vi "Restarts by Flow Sandbox Original (FPGA).vi"() -> ()   [LabVIEW 2019]
uses:
  <vilib>/eio/EIONode/EIONode.xnode
  <vilib>/rvi/eio/common/nirviEmuTemplateMethod_errors.vi
  <vilib>/rvi/FXPMathLib/FxpMul/XNode/nifxpmath_Multiplier.xnode
  <vilib>/rvi/FXPMathLib/sim/FxpSim.dll
  <vilib>/Platform/TimedLoop/XDataNode/wakeup.ctl
  <vilib>/Platform/TimedLoop/XDataNode/XDNodeRunTimeDep.lvlib
  <vilib>/Platform/TimedLoop/XDataNode/nitl_modes.ctl
  <vilib>/Platform/TimedLoop/XDataNode/timing_clust.ctl
  <vilib>/Platform/TimedLoop/XDataNode/XDataNode.xnode
  <vilib>/rvi/Analysis/measure/dc-rms/XNode/niFpgaDC-RMS.xnode
  <vilib>/rvi/DataTransferAndStorage/Container/XNode/niFpgaContainer.xnode
  <vilib>/rvi/FXPMathLib/FxpAdd/XNode/nifxpmath_Add.xnode
  <userlib>/_NI SPI IP/FPGA/Controllers/Public/Spi Master Inputs.ctl
  <vilib>/eio/EIOMethodNode/EIOMethodNode.xnode
  Controls/SPI Channels.ctl
  <vilib>/rvi/FIFO/Fifo_Resource/niFpgaFifoEmulationRefIn.vi
  <vilib>/rvi/interface/RandomDataEmulation/nirviRandomDataFpgaReadWriteTemplate.vi
  <vilib>/rvi/FXPMathLib/basic elements/FxpIntAccumulator/simVIs/DllFxpIntAccumulator_sub.vi
  <vilib>/rvi/FXPMathLib/basic elements/FxpIntAccumulator/XNode/nifxpmath_IntAccumulator.xnode
  <vilib>/rvi/FXPMathLib/FxpSqrt/XNode/nifxpmath_Sqrt.xnode
  <vilib>/rvi/Analysis/common/codeGenErrors/XNode/niFpgaXNodeCodeGenErrorHandle.vi
  <vilib>/rvi/FXPMathLib/FxpSqrt/simVIs/DllSqrtTemp_sub.vi
  <vilib>/fxp/LVFixedPointOverflowPolicyTypeDef.ctl
  <vilib>/rvi/FXPMathLib/FxpSqrt/subVIs/nifxpmath_Sqrt_SimConfig.ctl
  <vilib>/rvi/FXPMathLib/basic elements/FxpIntAccumulator/subVIs/nifxpmath_IntAccumulator_SimConfig.ctl
  <vilib>/rvi/FXPMathLib/FxpSub/XNode/nifxpmath_Sub.xnode
  <vilib>/rvi/Memory/Memory_Emulation/nirvimemoryFastEmulation.vi
  <vilib>/rvi/Memory/Memory_Emulation/nirvimemoryEmulation.vi
  <userlib>/_NI SPI IP/FPGA/Controllers/Public/Transfer Settings.ctl
panel:
  in  "Pres/Flow":bool
  out "DetPres Starts":u32
  out "Pressure":fxp<+/-,28,17>
  out "Flow":fxp<+/-,28,17>
  out "Current":fxp<+/-,28,17>
  out "DetFlow Starts":u32
  in  "Position":i32
  in  "PreDataPts":i32=2000
  in  "Reset Restarts":bool
  in  "AI24-31 Data to Write":u64 format="%.0x"
  out "AI24-31":fxp<+/-,28,17>[](array[numeric])
  out "Read Data 2":u64 format="%.0x"
  in  "AI24-31 Settings":T1 {"Direction Change Bit" max=64 step=1; "Transfer Length (bits)" min=1 max=64 step=1}
  out "AI16-23":fxp<+/-,28,17>[](array[numeric])
  in  "AI16-23 Data to Write":u64 format="%.0x"
  out "Read Data":u64 format="%.0x"
  in  "AI16-23 Settings":T1 {"Direction Change Bit" max=64 step=1; "Transfer Length (bits)" min=1 max=64 step=1}
  in  "AO0":fxp<+/-,20,5>
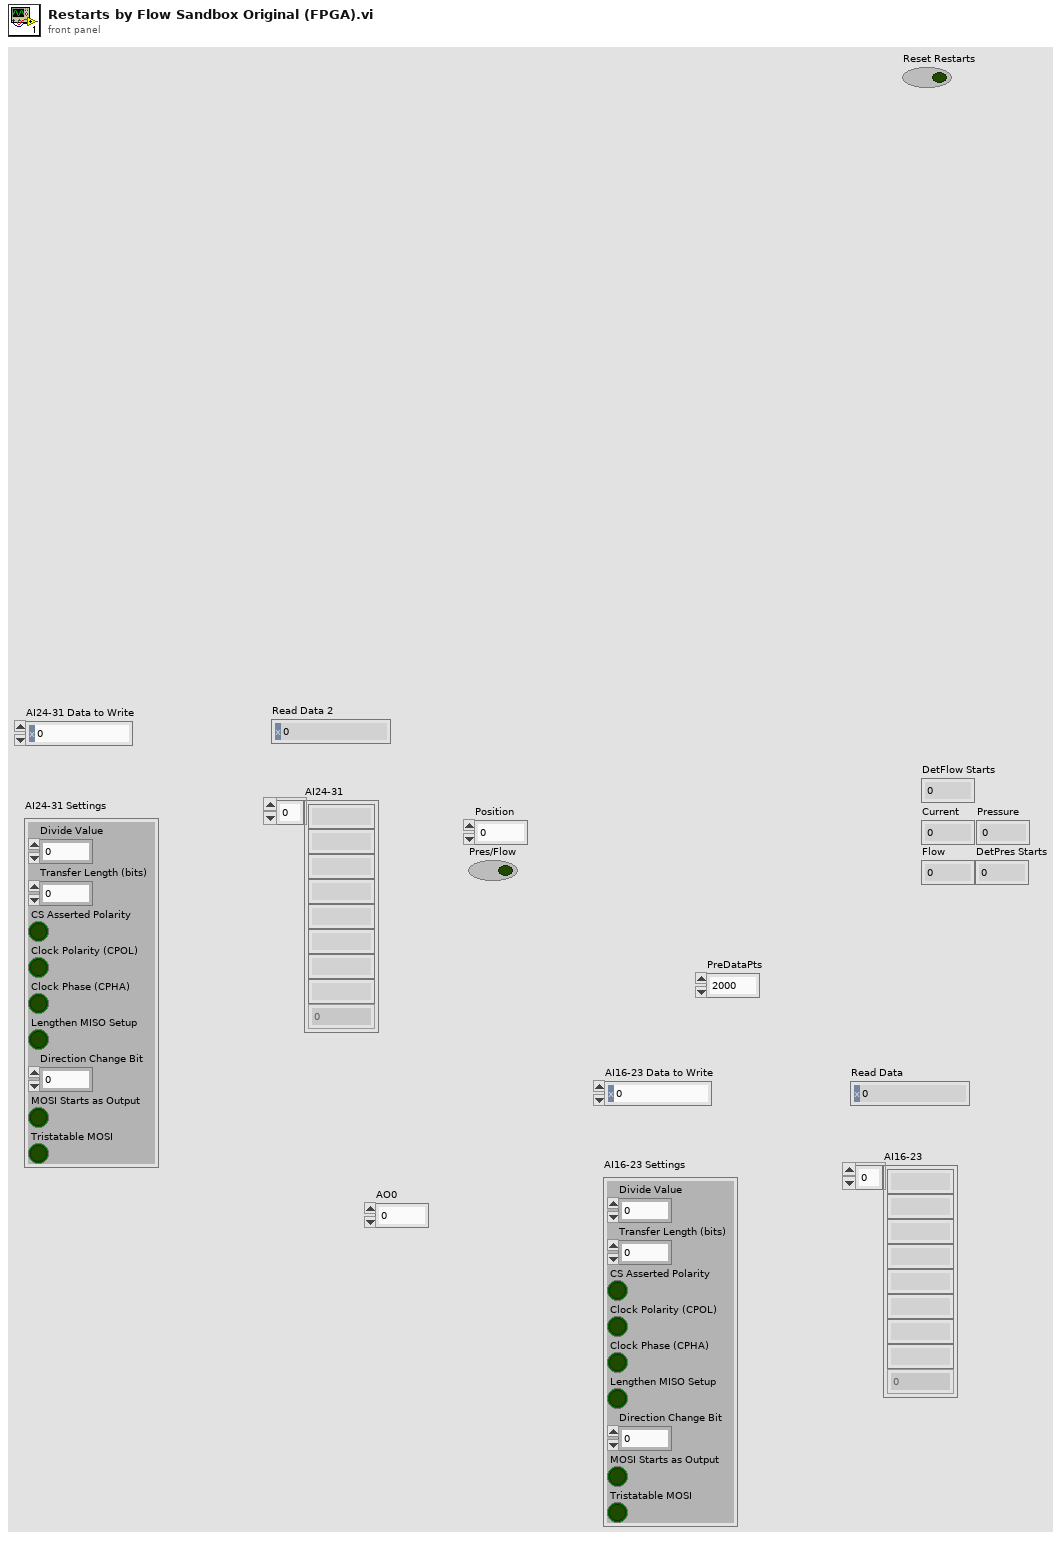
[diagram p1: front panel]
types:
  T1 = typedef "DIO SPI FPGA.lvlib/Transfer Settings.ctl" = cluster{"Divide Value":u8, "Transfer Length (bits)":u8, "CS Asserted Polarity":bool, "Clock Polarity (CPOL)":bool, "Clock Phase (CPHA)":bool, "Lengthen MISO Setup":bool, "Direction Change Bit":u8, "MOSI Starts as Output":bool, "Tristatable MOSI":bool}
  T2 = typedef "SPI Channels.ctl" = cluster{"CS":refnum<k21>, "CLK":refnum<k21>, "MOSI":refnum<k21>, "MISO":refnum<k21>}
  T3 = typedef "XDNodeRunTimeDep.lvlib/timing_clust.ctl" = cluster{"Expected End [f-1]":u64, "Actual End [f-1]":u64, "Finished Late? [f-1]":bool, "Expected End [i-1]":u64, "Actual End [i-1]":u64, "Finished Late? [i-1]":bool, "Expected Start [i]":u64, "Actual Start [i]":u64, "Expected Start [f]":u64, "Actual Start [f]":u64, "Source Name":string, "Structure Name":string, "Period":i64, "Deadline":i64, "Offset":i64, "Start":i64, "Priority":i32, "Timeout":i32, "Mode":T4, "Wakeup Reason":T5, "Error":errorcluster, "Source Type":string, "Secondary Source Type":string, "Global End Time":u64, "Global Start Time":u64, "Frame Duration":u64, "Iteration Duration":u64, "Assigned CPU":i32, "I/O Scan Engine Mode":u32}
  T4 = typedef "XDNodeRunTimeDep.lvlib/nitl_modes.ctl" = enum32{"No Change", "Process missed periods, maintain original phase", "Discard missed periods, maintain original phase", "Process missed periods, ignore original phase", "Discard missed periods, ignore original phase"}
  T5 = typedef "XDNodeRunTimeDep.lvlib/wakeup.ctl" = enum32{"Normal", "Aborted", "Asynchronous wakeup", "Timing source error", "Timed loop error", "Timeout"}
  T6 = typedef "DIO SPI FPGA.lvlib/Spi Master Inputs.ctl" = cluster{"MISO":bool}
  T7 = typedef "DIO SPI FPGA.lvlib/Spi Master Outputs.ctl" = cluster{"Chip Select":bool, "Clock":bool, "MOSI":bool, "MOSI OE":bool}
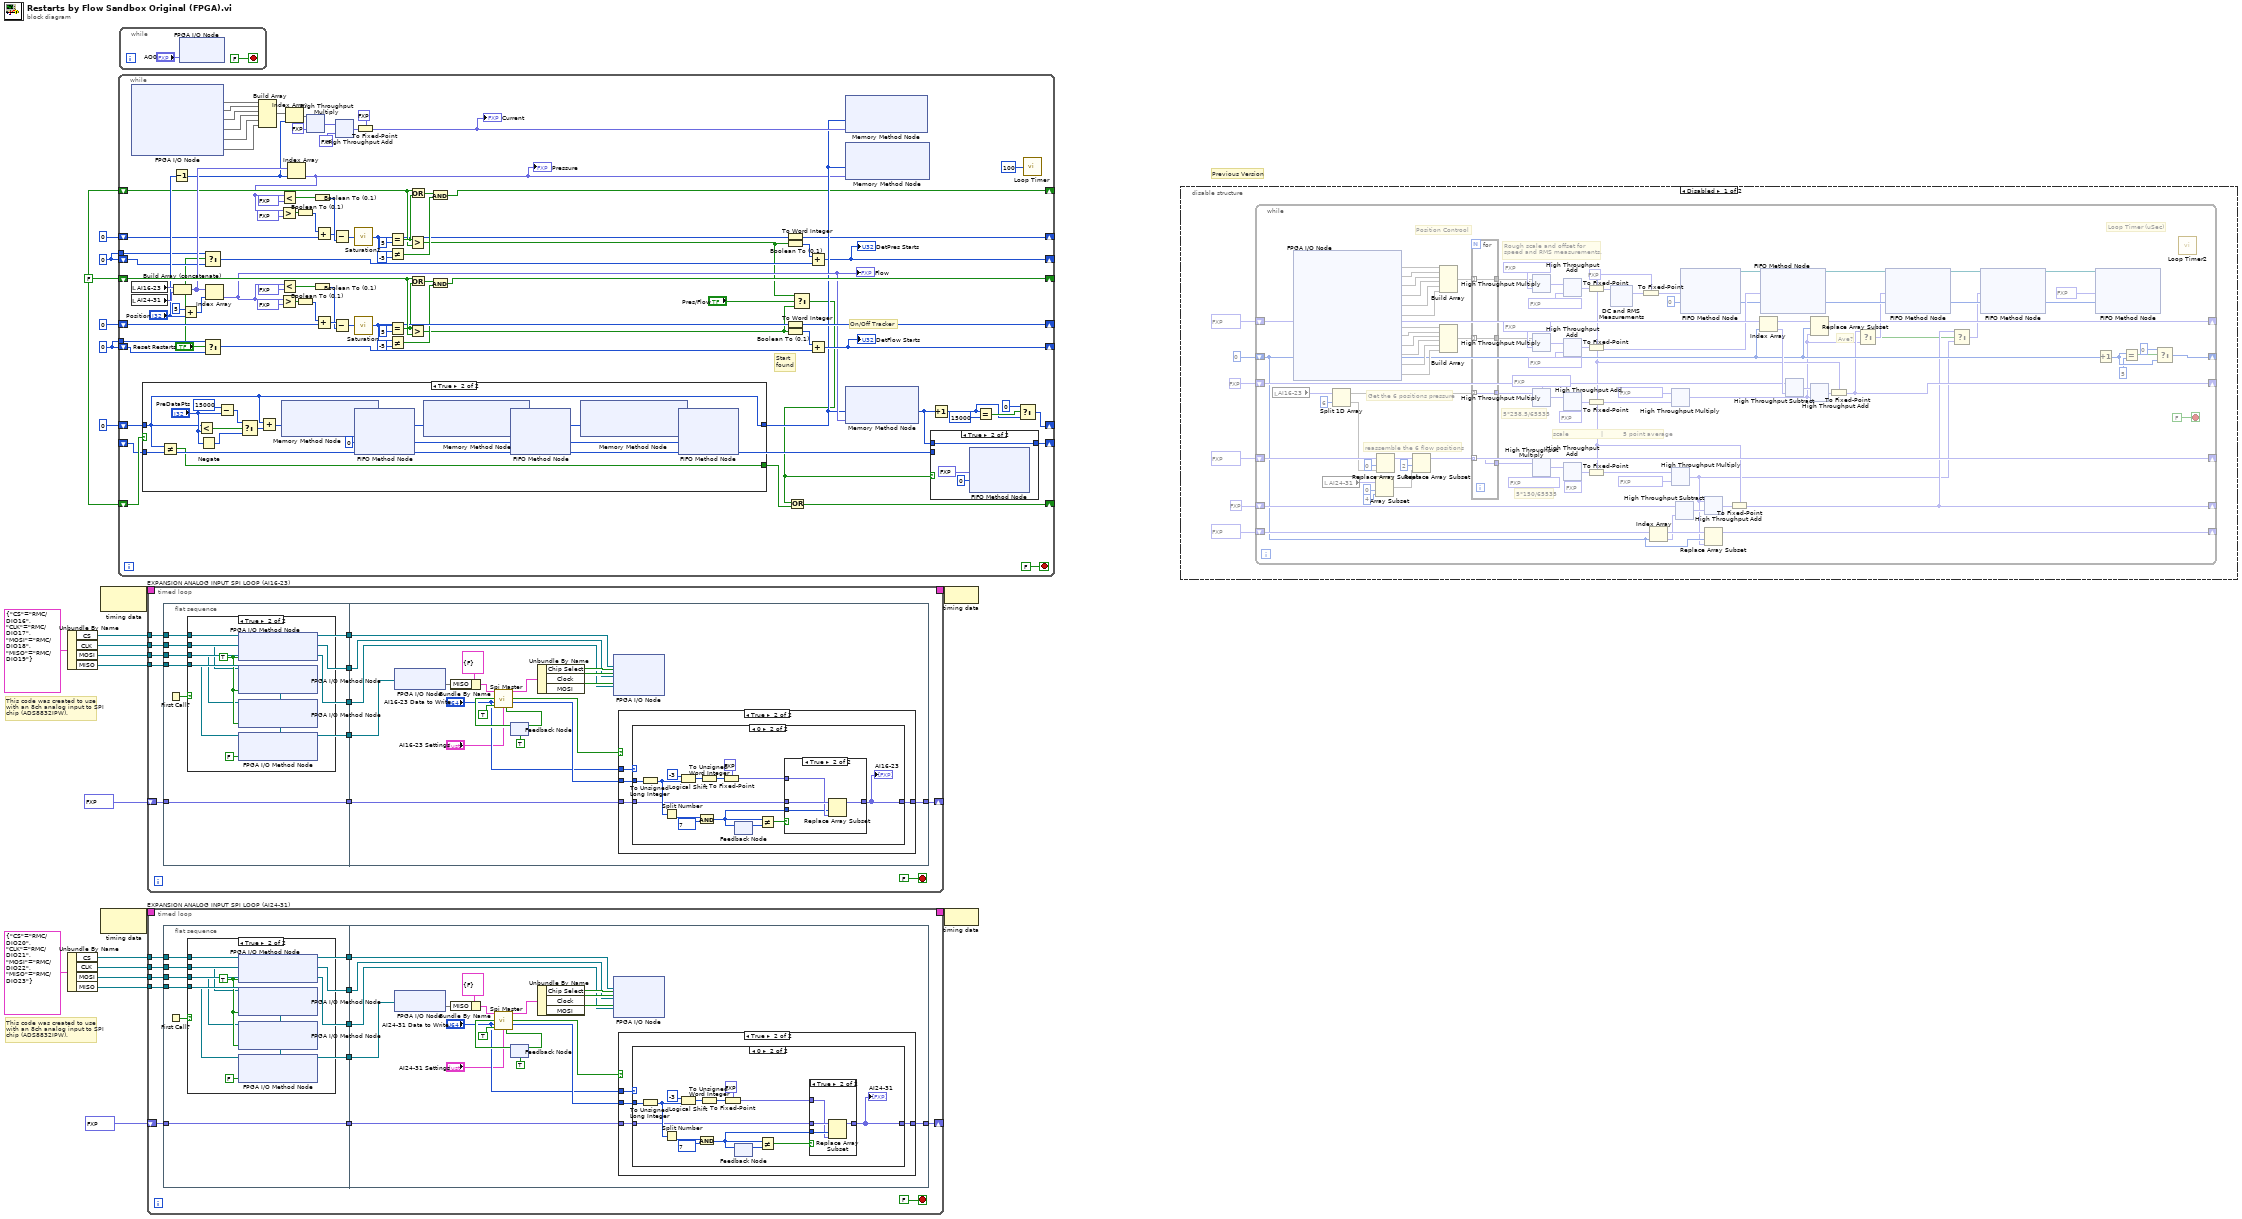
[diagram p0: block diagram]
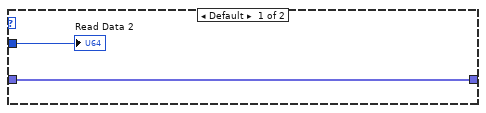
[diagram p7: hidden frame]
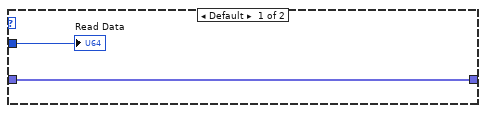
[diagram p11: hidden frame]
diagram:
  w1 = u32 0
  w4 = u32 0
  w3 = FALSE
  # "Previous Version"
  # "This code was created to use\nwith an 8ch analog input to SPI\nchip (ADS8832IPW)."
  # "This code was created to use\nwith an 8ch analog input to SPI\nchip (ADS8832IPW)."
  n1 = Unbundle By Name(T2 {"CS"="RMC/DIO16", "CLK"="RMC/DIO17", "MOSI"="RMC/DIO18", "MISO"="RMC/DIO19"} ("SPI Channels")) -> ("CS"=w16:refnum<k21>, "CLK"=w17:refnum<k21>, "MOSI"=w18:refnum<k21>, "MISO"=w19:refnum<k21>)
  n2 = Unbundle By Name(T2 {"CS"="RMC/DIO20", "CLK"="RMC/DIO21", "MOSI"="RMC/DIO22", "MISO"="RMC/DIO23"} ("SPI Channels")) -> ("CS"=w8:refnum<k21>, "CLK"=w9:refnum<k21>, "MOSI"=w10:refnum<k21>, "MISO"=w11:refnum<k21>)
  n3 = node-c288() -> (w22:T3)  [unwired: 1 in]
  n4 = node-c288() -> (w14:T3)  [unwired: 1 in]
  n5 = while {
    shift-right: [w72] -> _
    shift-left: w4 -> [w106]
    shift-right: [w107] -> _
    shift-left: w3 -> [w108]
    shift-right: [w104] -> _
    shift-left: i16 0 -> [w109]
    tunnel: w4 -> [w105]
    shift-right: [w96] -> _
    shift-left: 0 ("Address") -> [w95]
    shift-right: [w93] -> _
    shift-left: w3 -> [w91]
    shift-right: [w94] -> _
    shift-left: _ -> [w70]
    shift-right: [w33] -> _
    shift-left: w3 -> [w38]
    shift-right: [w34] -> _
    shift-left: i16 0 -> [w37]
    shift-right: [w35] -> _
    shift-left: w1 -> [w31]
    tunnel: w1 -> [w30]
    stop <- FALSE stop-if-true
    # "Start\nfound"
    # "On/Off Tracker"
    n6 = xnode "FPGA I/O Node"() -> ("Speed_Current_1 (AI0)"=w57, "Speed_Current_2 (AI1)"=w62, "Speed_Current_3 (AI2)"=w61, "Speed_Current_4 (AI3)"=w60, "Speed_Current_5 (AI4)"=w59, "Speed_Current_6 (AI5)"=w58)  [unwired: 6 in, 6 out]
    n7 = local read "AI16-23"() -> (w102:fxp<+/-,28,17>[])
    n8 = local read "AI24-31"() -> (w103:fxp<+/-,28,17>[])
    n9 = case shown="True" w91 {
      selector: w91 -> [w116 _]
      tunnel: w95 -> [w115 w121]
      tunnel: w70 -> [_ w123]
      tunnel: [w116 w122] -> w92
      tunnel: [w115 w121] -> w52
      frame False {
      }
      frame True {
        w118 = 0 ("Timeout")
        n10 = Not Equal?(x=w121, y=w123) -> (x != y?=w122:bool)
        n11 = Less?(x=w121, y="PreDataPts") -> (x < y?=w130:bool)
        n12 = Negate(x="PreDataPts") -> (-x=w127:i32)
        n13 = Subtract(x=15000 ("t"), y="PreDataPts") -> (x-y=w124:i32)
        n14 = Select(t=w124, s=w130, f=w127) -> (s? t:f=w129:i32)
        n15 = Add(x=w121, y=w129) -> (x+y=w119:i32)
        n16 = xnode ("Memory Method Node")("Address"=w119) -> ("Data"=w128:fxp<+/-,28,17>)  [unwired: 1 in, 1 out]
        n17 = xnode ("FIFO Method Node")("Element"=w128, "Timeout"=w118) -> ()  [unwired: 1 in, 2 out]
        n18 = xnode ("Memory Method Node")("Address"=w119) -> ("Data"=w120:fxp<+/-,28,17>)  [unwired: 1 in, 1 out]
        n19 = xnode ("FIFO Method Node")("Element"=w120, "Timeout"=w118) -> ()  [unwired: 1 in, 2 out]
        n20 = xnode ("Memory Method Node")("Address"=w119) -> ("Data"=w117:fxp<+/-,28,17>)  [unwired: 1 in, 1 out]
        n21 = xnode ("FIFO Method Node")("Element"=w117, "Timeout"=w118) -> ()  [unwired: 1 in, 2 out]
      }
    }
    n22 = Decrement(x="Position") -> (x-1=w53:i32)
    n23 = Build Array (concatenate)(w102, w103) -> (w54:fxp<+/-,28,17>[])
    n24 = Add(x=5 ("index"), y="Position") -> (x+y=w88:i32)
    n25 = Select(t=w30, s="Reset Restarts", f=w31) -> (s? t:f=w32:u32)
    n26 = Select(t=w105, s="Reset Restarts", f=w106) -> (s? t:f=w110:u32)
    n27 = Index Array(array=w54, index=w88) -> (element=w71:fxp<+/-,28,17>)
    "Flow" <- w71
    n28 = Build Array(w57, w62, w61, w60, w59, w58) -> (w63:void[])
    n29 = Greater?(x=w71, y=fxp<+/-,28,17> 13413.0) -> (0:w79:bool)
    n30 = Less?(x=w71, y=fxp<+/-,28,17> 13238.0) -> (x < y?=w80:bool)
    n31 = Index Array(array=w63, index=w53) -> (element=w69)
    n32 = Index Array(array=w54, index=w53) -> (element=w28:fxp<+/-,28,17>)
    "Pressure" <- w28
    n33 = Greater?(x=w28, y=fxp<+/-,28,17> 13413.0) -> (0:w46:bool)
    n34 = Less?(x=w28, y=fxp<+/-,28,17> 13238.0) -> (x < y?=w45:bool)
    n35 = Boolean To (0,1)(Boolean=w46) -> (0, 1=w50:i16)
    n36 = Boolean To (0,1)(Boolean=w79) -> (0, 1=w74:i16)
    n37 = xnode ("High Throughput Multiply")("x"=w69, "y"=fxp<+,5,5> 24.0 ("Current Scale")) -> ("x*y"=w66:fxp<+/-,29,10>)
    n38 = Boolean To (0,1)(Boolean=w45) -> (0, 1=w51:i16)
    n39 = Boolean To (0,1)(Boolean=w80) -> (0, 1=w73:i16)
    n40 = Add(x=w50, y=w37) -> (x+y=w41:i16)
    n41 = Add(x=w74, y=w109) -> (x+y=w84:i16)
    n42 = Subtract(x=w41, y=w51) -> (x-y=w42:i16)
    n43 = Subtract(x=w84, y=w73) -> (x-y=w83:i16)
    n44 = xnode ("High Throughput Add")("x"=w66, "y"=fxp<+/-,7,7> -60.0 ("Current Offset")) -> ("x+y"=w68:fxp<+/-,30,11>)
    n45 = call "Saturation2"("input"=w42) -> ("output"=w27:i32)  [unwired: 8 in]
    n46 = call "Saturation"("input"=w83) -> ("output"=w78:i32)  [unwired: 8 in]
    n47 = To Fixed-Point(fixed-point type=fxp<+/-,28,17> 0.0 ("out"), number=w68) -> (fixed-point=w56:fxp<+/-,28,17>)
    "Current" <- w56
    n48 = Equal?(x=w27, y=5) -> (x = y?=w47:bool)
    n49 = Not Equal?(x=w27, y=-5) -> (x != y?=w49:bool)
    n50 = Equal?(x=w78, y=5) -> (x = y?=w77:bool)
    n51 = Not Equal?(x=w78, y=-5) -> (x != y?=w75:bool)
    n52 = Greater?(x=w47, y=w38) -> (0:w25:bool)
    n53 = Greater?(x=w77, y=w108) -> (0:w24:bool)
    n54 = Or(x=w38, y=w47) -> (x .or. y?=w48:bool)
    n55 = Or(x=w108, y=w77) -> (x .or. y?=w76:bool)
    n56 = And(x=w48, y=w49) -> (x .and. y?=w33:bool)
    n57 = And(x=w76, y=w75) -> (x .and. y?=w107:bool)
    n58 = To Word Integer(number=w27) -> (16bit integer=w34:i16)
    n59 = Boolean To (0,1)(Boolean=w25) -> (0, 1=w36:i16)
    n60 = To Word Integer(number=w78) -> (16bit integer=w104:i16)
    n61 = Boolean To (0,1)(Boolean=w24) -> (0, 1=w85:i16)
    n62 = Select(t=w25, s="Pres/Flow", f=w24) -> (s? t:f=w23:bool)
    n63 = Or(x=w23, y=w92) -> (x .or. y?=w93:bool)
    n64 = Add(x=w36, y=w32) -> (x+y=w35:u32)
    "DetPres Starts" <- w35
    n65 = Add(x=w85, y=w110) -> (x+y=w72:u32)
    "DetFlow Starts" <- w72
    n66 = xnode ("Memory Method Node")("Address"=w52, "Data"=w56) -> ()  [unwired: 1 in, 1 out]
    n67 = xnode ("Memory Method Node")("Address"=w52, "Data"=w28) -> ()  [unwired: 1 in, 1 out]
    n68 = xnode ("Memory Method Node")("Address"=w52, "Data"=w71) -> ()  [unwired: 1 in, 1 out]
    n69 = case shown="True" w23 {
      tunnel: w52 -> [_ w112]
      tunnel: [w111 w112] -> w94
      tunnel: w70 -> [w111 _]
      frame False {
      }
      frame True {
        n70 = xnode ("FIFO Method Node")("Element"=fxp<+/-,28,17> -999.0, "Timeout"=0) -> ()  [unwired: 1 in, 2 out]
      }
    }
    n71 = Increment(x=w52) -> (x+1=w98:i32)
    n72 = Equal?(x=w98, y=15000) -> (x = y?=w99:bool)
    n73 = Select(t=0, s=w99, f=w98) -> (s? t:f=w96:i32)
    n74 = call "Loop Timer"("Count(uSec)"=u32 100 ("Loop Timer (uSec)")) -> ()  [unwired: 1 out]
  }
  n75 = while {
    stop <- FALSE stop-if-true
    n76 = xnode "FPGA I/O Node"("AO0"="AO0") -> ()  [unwired: 2 in, 2 out]
  }
  n77 = timed-loop "EXPANSION ANALOG INPUT SPI LOOP (AI16-23)" {
    timing: w22 -> [_]
    timing-out: [_] -> w21
    shift-right: [w141] -> _
    shift-left: fxp<+/-,28,17>[] [0.0, 0.0, 0.0, 0.0, 0.0, 0.0, 0.0, 0.0] -> [w142]
    tunnel: w16 -> [w140]
    tunnel: w17 -> [w139]
    tunnel: w18 -> [w138]
    tunnel: w19 -> [w137]
    stop <- FALSE stop-if-true
    n78 = flat-sequence {
      tunnel: [w149] -> w143
      tunnel: w142 -> [w149]
      tunnel: w140 -> [w148]
      tunnel: w139 -> [w147]
      tunnel: w138 -> [w146]
      tunnel: w137 -> [w145]
      tunnel: [w148] -> w136
      tunnel: [w147] -> w135
      tunnel: [w146] -> w134
      tunnel: [w145] -> w133
      tunnel: w143 -> [w163]
      tunnel: [w162] -> w141
      tunnel: w136 -> [w161]
      tunnel: w135 -> [w160]
      tunnel: w134 -> [w159]
      tunnel: w133 -> [w158]
      frame #0 {
        n79 = First Call?() -> (First Call?: T/F=w150:bool)
        n80 = case shown="True" w150 {
          tunnel: w148 -> [_ w154]
          tunnel: w147 -> [_ w153]
          tunnel: w146 -> [_ w152]
          tunnel: w145 -> [_ w151]
          frame False {
          }
          frame True {
            w156 = TRUE ("Enable")
            n81 = xnode "FPGA I/O Method Node"("FPGA I/O In"=w154, "Enable"=w156) -> ()  [unwired: 1 out]
            n82 = xnode "FPGA I/O Method Node"("FPGA I/O In"=w153, "Enable"=w156) -> ()  [unwired: 1 out]
            n83 = xnode "FPGA I/O Method Node"("FPGA I/O In"=w152, "Enable"=w156) -> ()  [unwired: 1 out]
            n84 = xnode "FPGA I/O Method Node"("FPGA I/O In"=w151, "Enable"=FALSE) -> ()  [unwired: 1 out]
          }
        }
      }
      frame #1 {
        n85 = xnode "FPGA I/O Node"("FPGA I/O In"=w158) -> ("I/O Item"=w171)  [unwired: 1 out]
        n86 = Bundle By Name(cluster=T6 {"MISO"=FALSE} ("spi input"), "MISO"=w171) -> (w172:T6)
        n87 = feedback #1(TRUE ("read data valid")) -> (w168:bool)
        n88 = call <userlib>:"Spi Master.vi"("spi input"=w172, "start strobe"=w168, "data to write"="AI16-23 Data to Write", "MOSI output enable done"=TRUE, "spi transfer settings"="AI16-23 Settings") -> ("spi output"=w177:T7, "read data valid"=w164:bool, "read data"=w169:u64, "ready for input"=w165:bool)  [unwired: 7 in]
        n89 = feedback-in #1(w165) -> ()
        n90 = Unbundle By Name(w177) -> ("Chip Select"=w176:bool, "Clock"=w175:bool, "MOSI"=w174:bool)
        n91 = xnode "FPGA I/O Node"("I/O Item"=w176, "FPGA I/O In"=w161, "I/O Item"=w175, "FPGA I/O In"=w160, "I/O Item"=w174, "FPGA I/O In"=w159) -> ()  [unwired: 3 out]
        n92 = case shown="True" w164 {
          tunnel: w169 -> [_ w182]
          tunnel: "AI16-23 Data to Write" -> [_ w181]
          tunnel: w163 -> [w178 w180]
          tunnel: [w178 w179] -> w162
          frame False {
          }
          frame True {
            n93 = case shown="0" w181 {
              tunnel: w182 -> [w184 w198]
              tunnel: w180 -> [w183 w191]
              tunnel: [w183 w190] -> w179
              frame Default {
                "Read Data" <- w184
              }
              frame 0 {
                n94 = To Unsigned Long Integer(number=w198) -> (unsigned 32bit integer=w192:u32)
                n95 = Split Number(x=w192) -> (lo(x)=w196:u16)  [unwired: 1 out]
                n96 = Logical Shift(y=i16 -3, x=w192) -> (x << y=w193:u32)
                n97 = And(x=w196, y=u16 7) -> (x .and. y?=w188:u16)
                n98 = To Unsigned Word Integer(number=w193) -> (unsigned 16bit integer=w186:u16)
                n99 = To Fixed-Point(fixed-point type=fxp<+/-,28,17> 0.0 ("AI0"), number=w186) -> (fixed-point=w185:fxp<+/-,28,17>)
                n100 = feedback #2() -> (w197:u16)  [unwired: 1 in]
                n101 = feedback-in #2(w188) -> ()
                n102 = Not Equal?(x=w188, y=w197) -> (x != y?=w189:bool)
                n103 = case shown="True" w189 {
                  tunnel: w191 -> [w199 w203]
                  tunnel: [w199 w202] -> w190
                  tunnel: w188 -> [_ w200]
                  tunnel: w185 -> [_ w201]
                  frame False {
                  }
                  frame True {
                    n104 = Replace Array Subset(array=w203, new element=w201, index=w200) -> (w202:fxp<+/-,28,17>[])
                  }
                }
                "AI16-23" <- w190
              }
            }
          }
        }
      }
    }
  }
  n105 = timed-loop "EXPANSION ANALOG INPUT SPI LOOP (AI24-31)" {
    timing: w14 -> [_]
    timing-out: [_] -> w13
    shift-right: [w214] -> _
    shift-left: fxp<+/-,28,17>[] [0.0, 0.0, 0.0, 0.0, 0.0, 0.0, 0.0, 0.0] -> [w215]
    tunnel: w8 -> [w213]
    tunnel: w9 -> [w212]
    tunnel: w10 -> [w211]
    tunnel: w11 -> [w210]
    stop <- FALSE stop-if-true
    n106 = flat-sequence {
      tunnel: [w222] -> w216
      tunnel: w215 -> [w222]
      tunnel: w213 -> [w221]
      tunnel: w212 -> [w220]
      tunnel: w211 -> [w219]
      tunnel: w210 -> [w218]
      tunnel: [w221] -> w209
      tunnel: [w220] -> w208
      tunnel: [w219] -> w207
      tunnel: [w218] -> w206
      tunnel: w216 -> [w236]
      tunnel: [w235] -> w214
      tunnel: w209 -> [w234]
      tunnel: w208 -> [w233]
      tunnel: w207 -> [w232]
      tunnel: w206 -> [w231]
      frame #0 {
        n107 = First Call?() -> (First Call?: T/F=w223:bool)
        n108 = case shown="True" w223 {
          tunnel: w221 -> [_ w227]
          tunnel: w220 -> [_ w226]
          tunnel: w219 -> [_ w225]
          tunnel: w218 -> [_ w224]
          frame False {
          }
          frame True {
            w229 = TRUE ("Enable")
            n109 = xnode "FPGA I/O Method Node"("FPGA I/O In"=w227, "Enable"=w229) -> ()  [unwired: 1 out]
            n110 = xnode "FPGA I/O Method Node"("FPGA I/O In"=w226, "Enable"=w229) -> ()  [unwired: 1 out]
            n111 = xnode "FPGA I/O Method Node"("FPGA I/O In"=w225, "Enable"=w229) -> ()  [unwired: 1 out]
            n112 = xnode "FPGA I/O Method Node"("FPGA I/O In"=w224, "Enable"=FALSE) -> ()  [unwired: 1 out]
          }
        }
      }
      frame #1 {
        n113 = xnode "FPGA I/O Node"("FPGA I/O In"=w231) -> ("I/O Item"=w244)  [unwired: 1 out]
        n114 = Bundle By Name(cluster=T6 {"MISO"=FALSE} ("spi input"), "MISO"=w244) -> (w245:T6)
        n115 = feedback #3(TRUE ("read data valid")) -> (w241:bool)
        n116 = call <userlib>:"Spi Master.vi"("spi input"=w245, "start strobe"=w241, "data to write"="AI24-31 Data to Write", "MOSI output enable done"=TRUE, "spi transfer settings"="AI24-31 Settings") -> ("spi output"=w250:T7, "read data valid"=w237:bool, "read data"=w242:u64, "ready for input"=w238:bool)  [unwired: 7 in]
        n117 = feedback-in #3(w238) -> ()
        n118 = Unbundle By Name(w250) -> ("Chip Select"=w249:bool, "Clock"=w248:bool, "MOSI"=w247:bool)
        n119 = xnode "FPGA I/O Node"("I/O Item"=w249, "FPGA I/O In"=w234, "I/O Item"=w248, "FPGA I/O In"=w233, "I/O Item"=w247, "FPGA I/O In"=w232) -> ()  [unwired: 3 out]
        n120 = case shown="True" w237 {
          tunnel: w242 -> [_ w255]
          tunnel: "AI24-31 Data to Write" -> [_ w254]
          tunnel: w236 -> [w251 w253]
          tunnel: [w251 w252] -> w235
          frame False {
          }
          frame True {
            n121 = case shown="0" w254 {
              tunnel: w255 -> [w257 w271]
              tunnel: w253 -> [w256 w264]
              tunnel: [w256 w263] -> w252
              frame Default {
                "Read Data 2" <- w257
              }
              frame 0 {
                n122 = To Unsigned Long Integer(number=w271) -> (unsigned 32bit integer=w265:u32)
                n123 = Split Number(x=w265) -> (lo(x)=w269:u16)  [unwired: 1 out]
                n124 = Logical Shift(y=i16 -3, x=w265) -> (x << y=w266:u32)
                n125 = And(x=w269, y=u16 7) -> (x .and. y?=w261:u16)
                n126 = To Unsigned Word Integer(number=w266) -> (unsigned 16bit integer=w259:u16)
                n127 = To Fixed-Point(fixed-point type=fxp<+/-,28,17> 0.0 ("AI0"), number=w259) -> (fixed-point=w258:fxp<+/-,28,17>)
                n128 = feedback #4() -> (w270:u16)  [unwired: 1 in]
                n129 = feedback-in #4(w261) -> ()
                n130 = Not Equal?(x=w261, y=w270) -> (x != y?=w262:bool)
                n131 = case shown="True" w262 {
                  tunnel: w264 -> [w272 w276]
                  tunnel: [w272 w275] -> w263
                  tunnel: w261 -> [_ w274]
                  tunnel: w258 -> [_ w273]
                  frame False {
                  }
                  frame True {
                    n132 = Replace Array Subset(array=w276, new element=w273, index=w274) -> (w275:fxp<+/-,28,17>[])
                  }
                }
                "AI24-31" <- w263
              }
            }
          }
        }
      }
    }
  }
  n133 = node-c288(w21) -> ()
  n134 = node-c288(w13) -> ()
  n135 = disable-structure shown="Disabled" {
    frame Disabled {
      n136 = while {
        shift-right: [w337] -> _
        shift-left: fxp<+/-,28,17>[] [0.0, 0.0, 0.0, 0.0, 0.0] -> [w331]
        shift-right: [w332] -> _
        shift-left: 0 -> [w297]
        shift-right: [w291] -> _
        shift-left: fxp<+/-,28,17> 0.0 -> [w326]
        shift-right: [w312] -> _
        shift-left: fxp<+/-,28,17>[] [0.0, 0.0, 0.0, 0.0, 0.0, 0.0] -> [w321]
        shift-right: [w298] -> _
        shift-left: fxp<+/-,28,17>[] [0.0, 0.0, 0.0, 0.0, 0.0] -> [w302]
        shift-right: [w289] -> _
        shift-left: fxp<+/-,28,17> 0.0 ("AI0") -> [w300]
        stop <- FALSE stop-if-true
        w292 = 0 ("Timeout")
        w294 = fxp<+/-,28,17> 0.0 ("out")
        # "Loop Timer (uSec)"
        # "Ave?"
        # "Position Controol"
        # "scale                |          5 point average"
        # "5*150/65535"
        # "reassemble the 6 flow positions"
        # "Get the 6 positions pressure"
        # "5*258.5/65535"
        # "Rough scale and offset for\nspeed and RMS measurements."
        n137 = local read "AI16-23"() -> (w324:fxp<+/-,28,17>[])
        n138 = xnode "FPGA I/O Node"() -> ("Speed_Current_1 (AI0)"=w368, "Speed_Current_2 (AI1)"=w374, "Speed_Current_3 (AI2)"=w373, "Speed_Current_4 (AI3)"=w372, "Speed_Current_5 (AI4)"=w371, "Speed_Current_6 (AI5)"=w370, "Controller_Current_1 (AI6)"=w358, "Controller_Current_2 (AI7)"=w357, "Controller_Current_3 (AI8)"=w356, "Controller_Current_4 (AI9)"=w355, "Controller_Current_5 (AI10)"=w354, "Controller_Current_6 (AI11)"=w353)  [unwired: 12 in, 12 out]
        n139 = local read "AI24-31"() -> (w319:fxp<+/-,28,17>[])
        n140 = Split 1D Array(array=w324, index=6) -> (first subarray=w322:fxp<+/-,28,17>[], second subarray=w313:fxp<+/-,28,17>[])
        n141 = Array Subset(array=w319, index=0, length=4) -> (w317:fxp<+/-,28,17>[])
        n142 = Replace Array Subset(array=w321, new element=w313, index=0) -> (w320:fxp<+/-,28,17>[])
        n143 = Replace Array Subset(array=w320, new element=w317, index=2) -> (w312:fxp<+/-,28,17>[])
        n144 = Build Array(w368, w374, w373, w372, w371, w370) -> (w366:void[])
        n145 = Build Array(w358, w357, w356, w355, w354, w353) -> (w367:void[])
        n146 = for {
          N: [_] -> w359
          tunnel: w367 -> [w485] mode=indexing
          tunnel: w322 -> [w484] mode=indexing
          tunnel: w366 -> [w486] mode=indexing
          tunnel: [w486] -> w360
          tunnel: [w485] -> w349
          tunnel: [w484] -> w344
          tunnel: w312 -> [w483] mode=indexing
          tunnel: [w483] -> w308
        }
        n147 = xnode ("High Throughput Multiply")("x"=w360, "y"=fxp<+,16,5> 24.0380859375 ("Current Scale")) -> ("x*y"=w365:fxp<+/-,40,10>)
        n148 = xnode ("High Throughput Multiply")("x"=w349, "y"=fxp<+,16,5> 24.0380859375 ("Current Scale")) -> ("x*y"=w352:fxp<+/-,40,10>)
        n149 = xnode ("High Throughput Multiply")("x"=w344, "y"=fxp<+,20,6> 0.01971435546875 ("Current Scale")) -> ("x*y"=w345:fxp<+/-,48,23>)
        n150 = xnode ("High Throughput Multiply")("x"=w308, "y"=fxp<+,20,6> 0.011474609375) -> ("x*y"=w307:fxp<+/-,48,23>)
        n151 = xnode ("High Throughput Add")("x"=w365, "y"=fxp<+/-,18,7> -60.09521484375 ("Current Offset")) -> ("x+y"=w361:fxp<+/-,41,11>)
        n152 = xnode ("High Throughput Add")("x"=w352, "y"=fxp<+/-,18,7> -60.09521484375 ("Current Offset")) -> ("x+y"=w348:fxp<+/-,41,11>)
        n153 = xnode ("High Throughput Add")("x"=w345, "y"=fxp<+/-,21,10> -258.5 ("Current Offset")) -> ("x+y"=w343:fxp<+/-,49,24>)
        n154 = xnode ("High Throughput Add")("x"=w307, "y"=fxp<+/-,21,10> -150.0 ("Current Offset")) -> ("x+y"=w305:fxp<+/-,49,24>)
        n155 = To Fixed-Point(fixed-point type=w294, number=w361) -> (fixed-point=w362:fxp<+/-,28,17>)
        n156 = To Fixed-Point(fixed-point type=w294, number=w348) -> (fixed-point=w325:fxp<+/-,28,17>)
        n157 = To Fixed-Point(fixed-point type=w294, number=w343) -> (fixed-point=w295:fxp<+/-,28,17>)
        n158 = To Fixed-Point(fixed-point type=w294, number=w305) -> (fixed-point=w303:fxp<+/-,28,17>)
        n159 = xnode ("DC and RMS Measurements")("input data"=w362) -> ("RMS"=w339:fxp<+,28,17>)  [unwired: 1 in, 1 out]
        n160 = To Fixed-Point(fixed-point type=w294, number=w339) -> (fixed-point=w338:fxp<+/-,28,17>)
        n161 = Index Array(array=w302, index=w297) -> (element=w301:fxp<+/-,28,17>)
        n162 = xnode ("High Throughput Multiply")("x"=fxp<+,16,5> 0.2001953125 ("y"), "y"=w295) -> ("x*y"=w290:fxp<+/-,28,17>)
        n163 = xnode ("High Throughput Multiply")("x"=w303, "y"=fxp<+,16,5> 0.2001953125) -> ("x*y"=w288:fxp<+/-,28,17>)
        n164 = xnode "High Throughput Subtract"("x"=w300, "y"=w301) -> ("x-y"=w293:fxp<+/-,29,18>)
        n165 = xnode ("FIFO Method Node")("Element"=w338, "Timeout"=w292) -> ("FIFO Out"=w342:refnum<k21>)  [unwired: 1 in, 1 out]
        n166 = xnode ("High Throughput Add")("x"=w288, "y"=w293) -> ("x+y"=w299:fxp<+/-,30,19>)
        n167 = Replace Array Subset(array=w302, new element=w288, index=w297) -> (w298:fxp<+/-,28,17>[])
        n168 = To Fixed-Point(fixed-point type=w294, number=w299) -> (fixed-point=w289:fxp<+/-,28,17>)
        n169 = Index Array(array=w331, index=w297) -> (element=w330:fxp<+/-,28,17>)
        n170 = xnode ("FIFO Method Node")("Element"=w325, "Timeout"=w292, "FIFO In"=w342) -> ("FIFO Out"=w341:refnum<k21>)  [unwired: 1 out]
        n171 = xnode "High Throughput Subtract"("x"=w326, "y"=w330) -> ("x-y"=w329:fxp<+/-,29,18>)
        n172 = Replace Array Subset(array=w331, new element=w290, index=w297) -> (w337:fxp<+/-,28,17>[])
        n173 = xnode ("High Throughput Add")("x"=w329, "y"=w290) -> ("x+y"=w327:fxp<+/-,30,19>)
        n174 = To Fixed-Point(fixed-point type=w294, number=w327) -> (fixed-point=w291:fxp<+/-,28,17>)
        n175 = Select(t=w291, f=w290) -> (s=w285:bool, s? t:f=w286:fxp<+/-,28,17>)
        n176 = xnode ("FIFO Method Node")("Element"=w286, "Timeout"=w292, "FIFO In"=w341) -> ("FIFO Out"=w311:refnum<k21>)  [unwired: 1 out]
        n177 = Select(t=w289, s=w285, f=w288) -> (s? t:f=w287:fxp<+/-,28,17>)
        n178 = xnode ("FIFO Method Node")("Element"=w287, "Timeout"=w292, "FIFO In"=w311) -> ("FIFO Out"=w310:refnum<k21>)  [unwired: 1 out]
        n179 = xnode ("FIFO Method Node")("Element"=fxp<+/-,28,17> -9999.0 ("AI0"), "Timeout"=w292, "FIFO In"=w310) -> ()  [unwired: 2 out]
        n180 = Increment(x=w297) -> (x+1=w335:i32)
        n181 = Equal?(x=w335, y=5) -> (x = y?=w336:bool)
        n182 = Select(t=0, s=w336, f=w335) -> (s? t:f=w332:i32)
        n183 = call "Loop Timer2"() -> ("Count(uSec)"=w328:u32)  [unwired: 1 out]
      }
    }
    frame Enabled {
    }
  }
